vi "ClustertoRawString.vi"(8 "error in (no error)":errorcluster, 11 "DataOut":T1) -> (0 "error out":errorcluster, 3 "DataOut":string)   [LabVIEW 2017]
doc: "This VI converts the outbound data cluster 'Data Out' to a JSON string ready for transfer via UDP."
uses:
  TypeDefs/dataOut.ctl
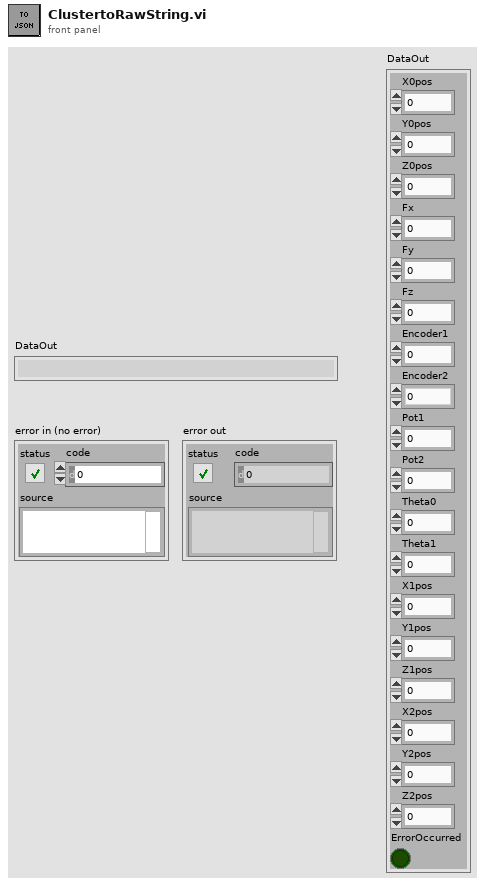
[diagram p1: front panel]
types:
  T1 = typedef "dataOut.ctl" = cluster{"X0pos":dbl, "Y0pos":dbl, "Z0pos":dbl, "Fx":dbl, "Fy":dbl, "Fz":dbl, "Encoder1":i32, "Encoder2":i32, "Pot1":dbl, "Pot2":dbl, "Theta0":dbl, "Theta1":dbl, "X1pos":dbl, "Y1pos":dbl, "Z1pos":dbl, "X2pos":dbl, "Y2pos":dbl, "Z2pos":dbl, "ErrorOccurred":bool}
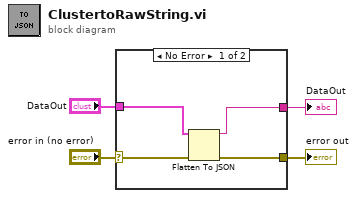
[diagram p0: block diagram]
diagram:
  n1 = case shown="No Error" "error in (no error)" {
    selector: "error in (no error)" -> [w8 w9]
    tunnel: [w7 w9] -> w3
    tunnel: "DataOut" -> [w6 _]
    tunnel: [w5 _] -> w1
    frame No Error {
      n2 = Flatten To JSON(anything=w6, error in (no error)=w8) -> (JSON string=w5:string, 11:w7:errorcluster)  [unwired: 1 in]
    }
    frame Error {
    }
  }
  "error out" <- w3
  "DataOut" <- w1
